vi "Main.vi"() -> ()   [LabVIEW 2011]
uses:
  ChM.ctl
panel:
  out "Результат":dbl(graph)
  in  "Exit":bool
  in  "Stop":bool
  in  "Почати генерацію чисел":bool
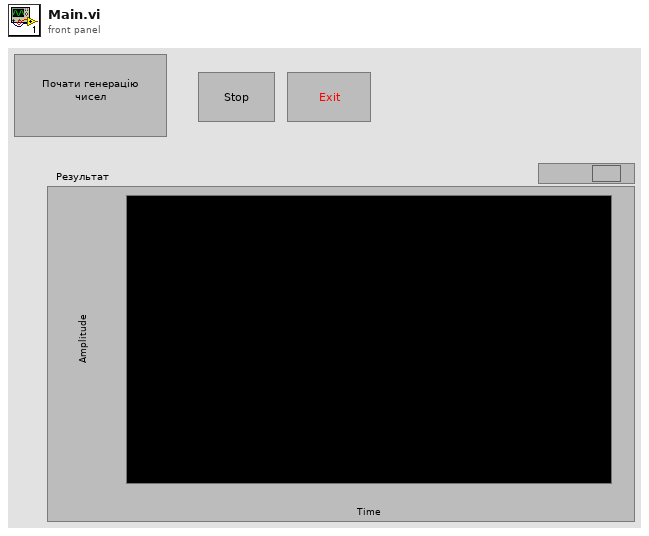
[diagram p1: front panel]
types:
  T1 = typedef "ChM.ctl" = enum16{"Gener", "Stop", "Exit"}
  T2 = enum32{"Invalid", "Standard", "Closed", "Hidden", "Minimized", "Maximized"}
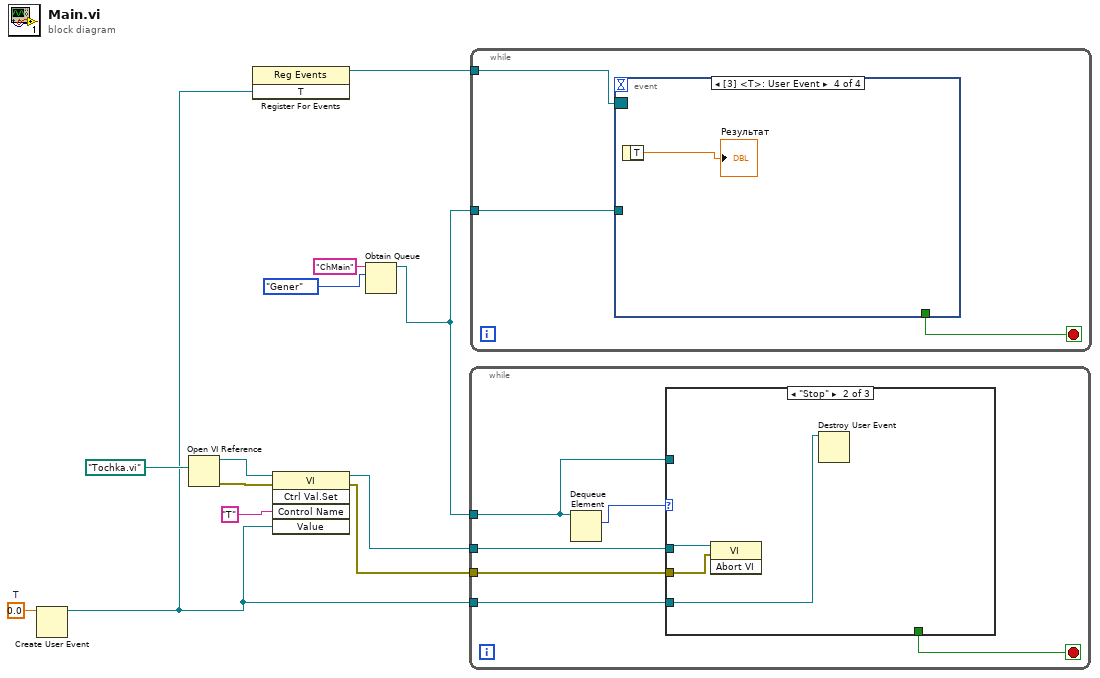
[diagram p0: block diagram]
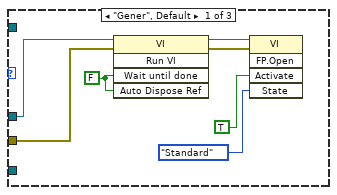
[diagram p2: hidden frame]
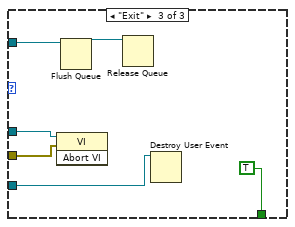
[diagram p3: hidden frame]
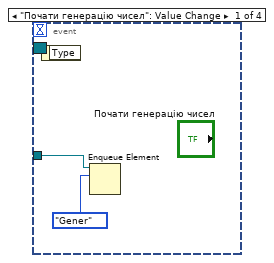
[diagram p4: hidden frame]
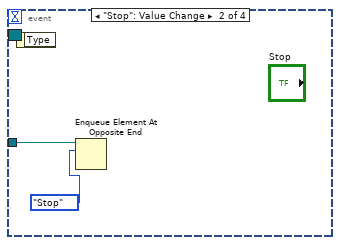
[diagram p5: hidden frame]
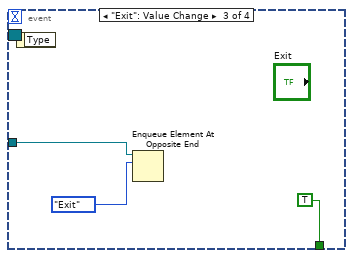
[diagram p6: hidden frame]
diagram:
  w4 = 0.0  # T
  n1 = Create User Event(user event datatype=w4) -> (user event=w1:refnum<user-event>)  [unwired: 1 in, 1 out]
  n2 = Open VI Reference(vi path=path "Tochka.vi") -> (vi reference=w10:refnum<vi>, error out=w9:errorcluster)  [unwired: 5 in]
  n3 = register-events(w1) -> (reference out=w3:refnum<event-registration>)  [unwired: 2 in, 1 out]
  n4 = invoke class="VI" method="Ctrl Val.Set"(reference=w10, error in=w9, "Control Name"="T", "Value"=w1) -> (reference out=w5:refnum<vi>, error out=w6:errorcluster)  [unwired: 1 in, 3 out]
  n5 = Obtain Queue(name (unnamed)="ChMain", element data type=ChM."Gener" ("Enum")) -> (queue out=w2:refnum<queue>)  [unwired: 3 in, 2 out]
  n6 = while {
    tunnel: w2 -> [w17]
    tunnel: w6 -> [w15]
    tunnel: w5 -> [w14]
    tunnel: w1 -> [w13]
    stop <- w16 stop-if-true
    n7 = Dequeue Element(queue=w17) -> (element=w18:T1)  [unwired: 2 in, 3 out]
    n8 = case shown="\"Stop\"" w18 {
      tunnel: w17 -> [_ _ w34]
      tunnel: [_ _ TRUE] -> w16
      tunnel: w15 -> [w19 w27 w30]
      tunnel: w14 -> [w20 w28 w31]
      tunnel: w13 -> [_ w26 w29]
      frame "Gener", Default {
        w25 = FALSE ("Wait Until Done")
        n9 = invoke class="VI" method="Run VI"(reference=w20, error in=w19, "Wait until done"=w25, "Auto Dispose Ref"=w25) -> (reference out=w24:refnum<vi>, error out=w23:errorcluster)  [unwired: 1 in, 3 out]
        n10 = invoke class="VI" method="FP.Open"(reference=w24, error in=w23, "Activate"=TRUE ("Activate?"), "State"=T2."Standard") -> ()  [unwired: 1 in, 5 out]
      }
      frame "Stop" {
        n11 = invoke class="VI" method="Abort VI"(reference=w28, error in=w27) -> ()  [unwired: 1 in, 3 out]
        n12 = Destroy User Event(user event=w26) -> ()  [unwired: 1 in, 1 out]
      }
      frame "Exit" {
        n13 = invoke class="VI" method="Abort VI"(reference=w31, error in=w30) -> ()  [unwired: 1 in, 3 out]
        n14 = Flush Queue(queue=w34) -> (queue out=w33:refnum<queue>)  [unwired: 1 in, 2 out]
        n15 = Release Queue(queue=w33) -> ()  [unwired: 2 in, 3 out]
        n16 = Destroy User Event(user event=w29) -> ()  [unwired: 1 in, 1 out]
      }
    }
  }
  n17 = while {
    tunnel: w2 -> [w37]
    tunnel: w3 -> [w35]
    stop <- w36 stop-if-true
    n18 = event shown="[3] <T>: User Event" {
      selector: w35 -> [_ _ _ _]
      dyn-events: _ -> [_ _ _ _]
      timeout: _ -> [_ _ _ _]
      tunnel: w37 -> [w39 w41 w44 _]
      tunnel: [_ _ TRUE _] -> w36
      event "Почати генерацію чисел": Value Change {
        n19 = event-data() -> ()  [unwired: 1 in, 1 out]
        n20 = Enqueue Element(queue=w39, element=ChM."Gener" ("Enum")) -> ()  [unwired: 2 in, 3 out]
      }
      event "Stop": Value Change {
        n21 = event-data() -> ()  [unwired: 1 in, 1 out]
        n22 = Enqueue Element At Opposite End(queue=w41, element=ChM."Stop" ("Enum")) -> ()  [unwired: 2 in, 3 out]
      }
      event "Exit": Value Change {
        n23 = event-data() -> ()  [unwired: 1 in, 1 out]
        n24 = Enqueue Element At Opposite End(queue=w44, element=ChM."Exit" ("Enum")) -> ()  [unwired: 2 in, 3 out]
      }
      event User Event {
        n25 = event-data() -> ("T"=→"Результат":dbl)  [unwired: 1 in]
      }
    }
  }
